vi "Shortcuts.vi"   [LabVIEW 2016]
uses:
  Instrument/Instrument.lvclass
  RemoteControl.STM/RemoteControl.STM.lvclass
  RemoteControl/RemoteControl.lvclass
  Logger.Error/Logger.Error.lvclass
  Logger/Logger.lvclass
  Configuration/Configuration.lvclass
  <vilib>/JKI/JKI SMO/SMO/SMO.lvclass
  <vilib>/JKI/JKI SMO/SMO.UI/SMO.UI.lvclass
  SCPI/SCPI.lvclass
  Instrument UI/Instrument UI.lvclass
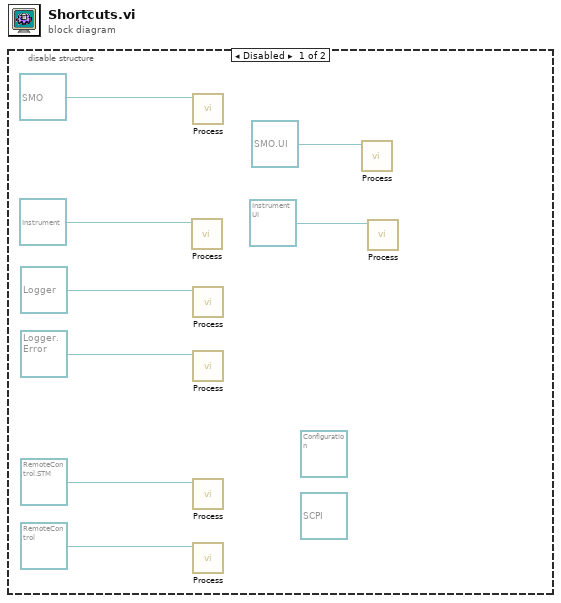
[diagram p0: block diagram]
diagram:
  n1 = disable-structure shown="Disabled" {
    frame Disabled {
      (unwired) refnum<class "SCPI.lvclass"> refnum ("SCPI.lvclass")
      (unwired) refnum<class "Configuration.lvclass"> refnum ("Configuration.lvclass")
      n2 = call-dynamic "Process.vi"("Instrument"=refnum<class "Instrument.lvclass"> refnum ("Instrument.lvclass")) -> ()  [unwired: 9 in, 2 out]
      n3 = call-dynamic "Process.vi"("SMO"=refnum<class "SMO.lvclass"> refnum) -> ()  [unwired: 9 in, 2 out]
      n4 = call-dynamic "Process.vi"("Logger"=refnum<class "Logger.lvclass"> refnum ("Logger.lvclass")) -> ()  [unwired: 9 in, 2 out]
      n5 = call-dynamic "Process.vi"("Logger.Error"=refnum<class "Logger.Error.lvclass"> refnum ("Logger.Error.lvclass")) -> ()  [unwired: 9 in, 2 out]
      n6 = call-dynamic "Process.vi"("RemoteControl"=refnum<class "RemoteControl.STM.lvclass"> refnum ("RemoteControl.STM.lvclass")) -> ()  [unwired: 9 in, 2 out]
      n7 = call-dynamic "Process.vi"("RemoteControl"=refnum<class "RemoteControl.lvclass"> refnum ("RemoteControl.lvclass")) -> ()  [unwired: 9 in, 2 out]
      n8 = call-dynamic "Process.vi"("SMO.UI"=refnum<class "SMO.UI.lvclass"> refnum) -> ()  [unwired: 9 in, 2 out]
      n9 = call-dynamic "Process.vi"("Instrument UI in"=refnum<class "Instrument UI.lvclass"> refnum ("Instrument UI.lvclass")) -> ()  [unwired: 9 in, 2 out]
    }
    frame Enabled {
    }
  }
